vi "Select Active BuildSpec.vi"(8 "error in (no error)":errorcluster, 9 "Build Spec Name in":string, 10 "Target Name in":string, 11 "Project Sync Tools in":refnum<class "Project Sync Tools.lvclass">) -> (0 "error out":errorcluster, 3 "Project Sync Tools out":refnum<class "Project Sync Tools.lvclass">)   [LabVIEW 2019, in "Project Sync Tools.lvclass"]
uses:
  Project Sync Tools.lvclass
  Project Sync Tools.lvclass/Project Sync Tools.ctl
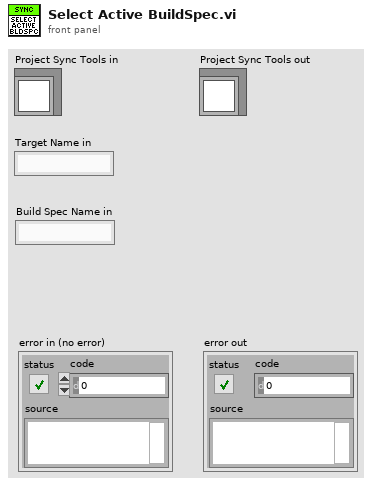
[diagram p1: front panel]
types:
  T1 = typedef "Project Sync Tools.lvclass/BuildSpec Parameters.ctl" = cluster{"BuildSpec Ref":refnum<vi>, "Target Name":string, "Build Spec Name":string, "Tags":string[], "Tag Values":variant[]}
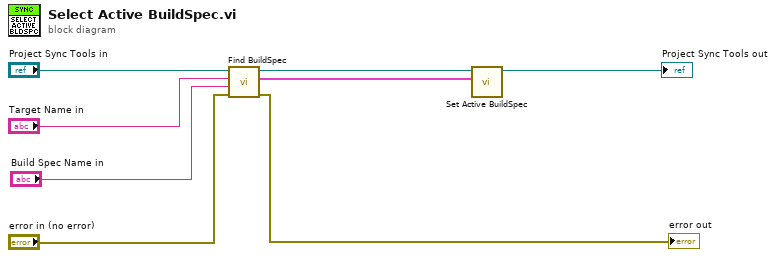
[diagram p0: block diagram]
diagram:
  n1 = call "Find BuildSpec.vi"("Error In"="error in (no error)", "Build Spec Name in"="Build Spec Name in", "Target Name in"="Target Name in", "Project Sync Tools in"="Project Sync Tools in") -> ("Error Out"=→"error out":errorcluster, "Build Spec out"=w3:T1, "Project Sync Tools out"=w4:refnum<class "Project Sync Tools.lvclass">)  [unwired: 4 in, 1 out]
  n2 = call "Set Active BuildSpec.vi"("Build Spec Parameters"=w3, "Project Sync Tools in"=w4) -> ("Project Sync Tools out"=→"Project Sync Tools out":refnum<class "Project Sync Tools.lvclass">)  [unwired: 9 in]
